vi "4431 Voltage Update.vi"(1 "4431 output":dbl(slide)=-0.0 min=-3.5 max=3.5 scale=-3.5..3.5, 8 "error in":errorcluster, 9 "Amplified output":dbl(slide) min=-50.0 max=50.0 scale=-45.0..45.0, 11 "Physical Channel(s)":tag="Dev2/ao0") -> (0 "error out":errorcluster)   [LabVIEW 2016]
doc: "This example demonstrates how to generate a finite amount of data from a buffer in your computer's memory."
uses:
  <vilib>/DAQmx/write.llb/DAQmx Write (Analog 1D DBL 1Chan NSamp).vi
  <vilib>/DAQmx/create/channels.llb/DAQmx Create Channel (AO-Voltage-Basic).vi
  <vilib>/DAQmx/configure/timing.llb/DAQmx Timing (Sample Clock).vi
  <vilib>/DAQmx/miscellaneous.llb/DAQmx Fill In Error Info.vi
  <resource>/objmgr/daqmx.rc
panel:
  in  "Amplifier Gain":dbl=-15.0 min=1.0
  in  "Max Voltage":dbl=3.5
  in  "Min Voltage":dbl=-3.5 min=-3.5 max=0.0
  # "Waveform Settings"
  # "Channel Settings"
  # "Instructions"
  # "-This VI will set a DC output to a NI USB-4431 DSA DAQ\n-The absolute limits are +/- 3.5 V\n- The voltage will be maintained even when the VI is not running & if LabVIEW is shutdown"
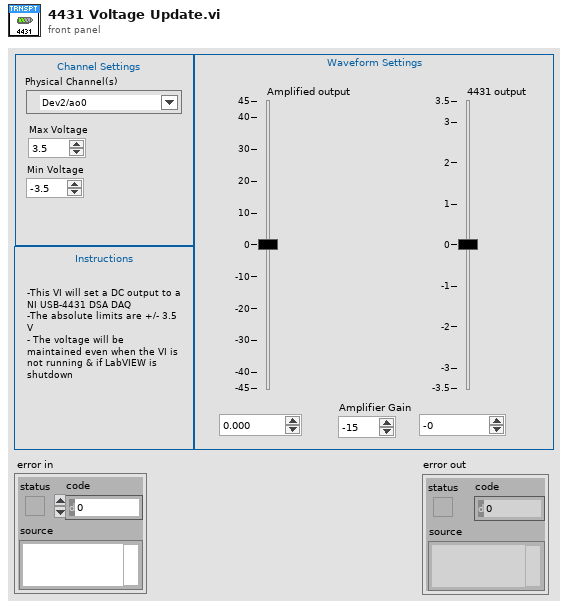
[diagram p1: front panel]
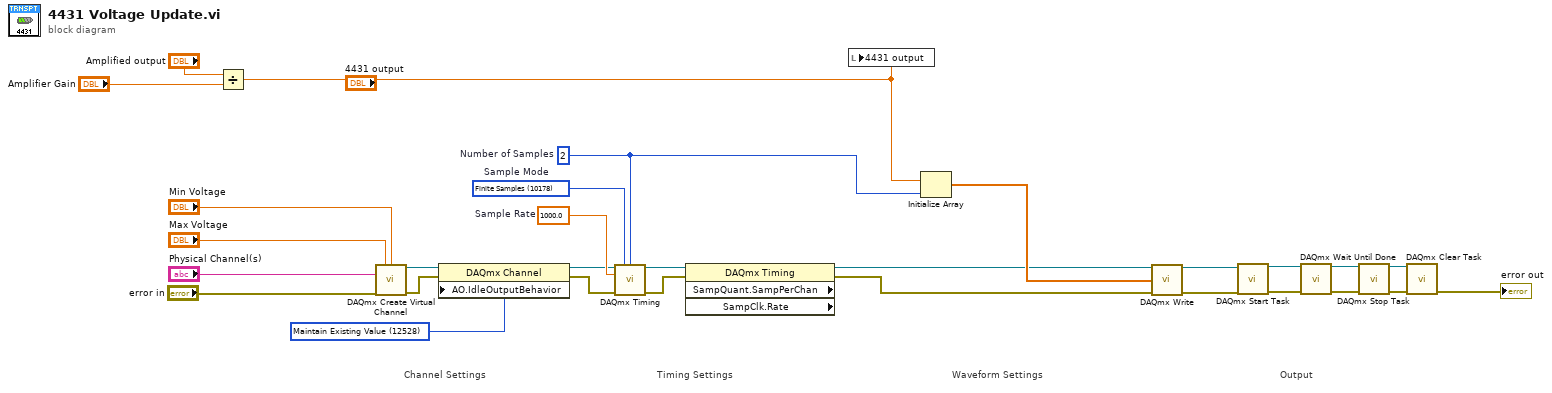
[diagram p0: block diagram]
diagram:
  w3 = 2  # Number of Samples
  w25 = 1000.0  # Sample Rate
  w11 = 12528 items=["Zero Volts"=12526, "High-Impedance"=12527, "Maintain Existing Value"=12528] ("AO.IdleOutputBehavior")
  w28 = 10178 items=["Finite Samples"=10178, "Continuous Samples"=10123, "Hardware Timed Single Point"=12522]  # Sample Mode
  # "Output"
  # "Waveform Settings"
  # "Timing Settings"
  # "Channel Settings"
  n1 = Divide(x="Amplified output", y="Amplifier Gain") -> (x/y=w4:dbl)
  n2 = call-poly <vilib>:"DAQmx Create Virtual Channel.vi"("maximum value"="Max Voltage", "minimum value"="Min Voltage", "physical channels"="Physical Channel(s)", "error in"="error in") -> ("task out"=w27:refnum<k21>, "error out"=w13:errorcluster)  [unwired: 10 in]
  n3 = property class="DAQmx Channel"(reference=w27, error in=w13, "AO.IdleOutputBehavior"=w11) -> (reference out=w14:refnum<k21>, error out=w12:errorcluster)
  n4 = call-poly <vilib>:"DAQmx Timing.vi"("task/channels in"=w14, "sample mode"=w28, "samples per channel"=w3, "rate"=w25, "error in"=w12) -> ("task out"=w29:refnum<k21>, "error out"=w9:errorcluster)  [unwired: 9 in]
  n5 = property class="DAQmx Timing" props=["SampQuant.SampPerChan", "SampClk.Rate"](reference=w29, error in=w9) -> (reference out=w1:refnum<k21>, error out=w10:errorcluster)  [unwired: 2 out]
  n6 = local write "4431 output"(w4) -> ()
  n7 = Initialize Array(w4, w3) -> (w2:dbl[])
  n8 = call-poly <vilib>:"DAQmx Write.vi"("task/channels in"=w1, "data"=w2, "error in"=w10) -> ("task out"=w22:refnum<k21>, "error out"=w21:errorcluster)  [unwired: 10 in, 1 out]
  n9 = call <vilib>:"DAQmx Start Task.vi"("task/channels in"=w22, "error in"=w21) -> ("task out"=w20:refnum<k21>, "error out"=w19:errorcluster)  [unwired: 12 in]
  n10 = call <vilib>:"DAQmx Wait Until Done.vi"("task/channels in"=w20, "error in"=w19) -> ("task out"=w16:refnum<k21>, "error out"=w15:errorcluster)  [unwired: 12 in]
  n11 = call <vilib>:"DAQmx Stop Task.vi"("task/channels in"=w16, "error in"=w15) -> ("task out"=w18:refnum<k21>, "error out"=w17:errorcluster)  [unwired: 12 in]
  n12 = call <vilib>:"DAQmx Clear Task.vi"("task in"=w18, "error in"=w17) -> ("error out"=→"error out":errorcluster)  [unwired: 13 in]
